vi "GLdrv_TRANS_OUTP_DATA.vi"(0 "Connection ID":T1, 5 "Start Byte":i32, 7 "End Byte":i32, 11 "error in (no error)":errorcluster, 13 "Query(f)":bool) -> (4 "Connection ID Out":T1, 10 "Data out":string, 15 "error out":errorcluster)   [LabVIEW 2017, in "GL860_Driver.lvlib"]
doc: "データ転送\nHEAD：　データヘッダ転送　（別紙参照）\n<NR1>,<NR1>：　開始点数、終了点数の設定\n例) TRANS:OUTP:DATA 1,100"
uses:
  GL860_Driver.lvlib
  ConnectionID.ctl
  GLdrv_RW.ctl
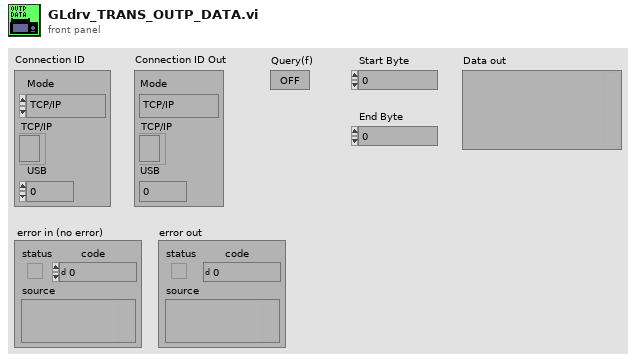
[diagram p1: front panel]
types:
  T1 = typedef "ConnectionID.ctl" = cluster{"Mode":enum16{"TCP/IP", "USB"}, "TCP/IP":refnum<k5>, "USB":i32}
  T2 = typedef "GLdrv_RW.ctl" = enum16{"Auto", "Read", "Write", "Buffer"}
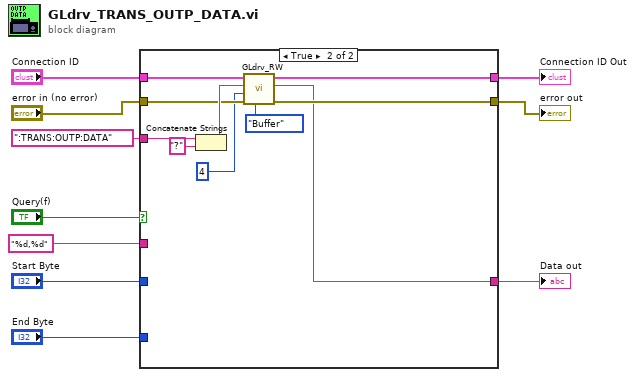
[diagram p0: block diagram]
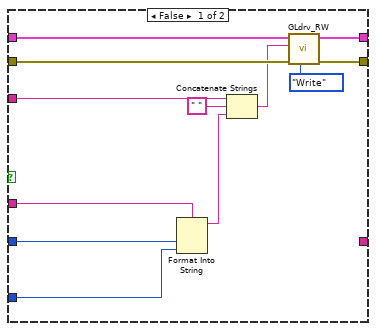
[diagram p2: hidden frame]
diagram:
  n1 = case shown="TRUE" "Query(f)" {
    tunnel: ":TRANS:OUTP:DATA" ("Command") -> [w22 w32]
    tunnel: [w17 w26] -> w10
    tunnel: [w19 w29] -> w9
    tunnel: "Connection ID" -> [w20 w30]
    tunnel: "error in (no error)" -> [w18 w27]
    tunnel: "Start Byte" -> [w13 _]
    tunnel: "%d,%d" ("Param") -> [w12 _]
    tunnel: [_ w25] -> w2
    tunnel: "End Byte" -> [w11 _]
    frame False {
      n2 = Format Into String(format string=w12, w13, w11) -> (resulting string=w14:string)  [unwired: 2 in, 1 out]
      n3 = Concatenate Strings(w22, " " ("string"), w14) -> (w16:string)
      n4 = call "GLdrv_RW.vi"("Mode(read)"=GLdrv_RW."Write", "error in (no error)"=w18, "data in"=w16, "Connection ID"=w20) -> ("error out"=w17:errorcluster, "Connection ID Out"=w19:T1)  [unwired: 3 in, 3 out]
    }
    frame True {
      n5 = Concatenate Strings(w32, "?" ("string")) -> (w28:string)
      n6 = call "GLdrv_RW.vi"("Mode(read)"=GLdrv_RW."Buffer", "error in (no error)"=w27, "Count(0:[CR+LF])"=u32 4, "data in"=w28, "Connection ID"=w30) -> ("error out"=w26:errorcluster, "data out"=w25:string, "Connection ID Out"=w29:T1)  [unwired: 2 in, 2 out]
    }
  }
  "Connection ID Out" <- w9
  "error out" <- w10
  "Data out" <- w2
